vi "Read ballPossession.vi"(8 "error in (no error)":errorcluster, 11 "Events in":refnum<class "Events.lvclass">) -> (0 "error out":errorcluster, 2 "Enum":T1, 3 "Events out":refnum<class "Events.lvclass">)   [LabVIEW 2023, in "Events.lvclass"]
uses:
  Events.lvclass
  Possession.ctl
  Events.lvclass/Events.ctl
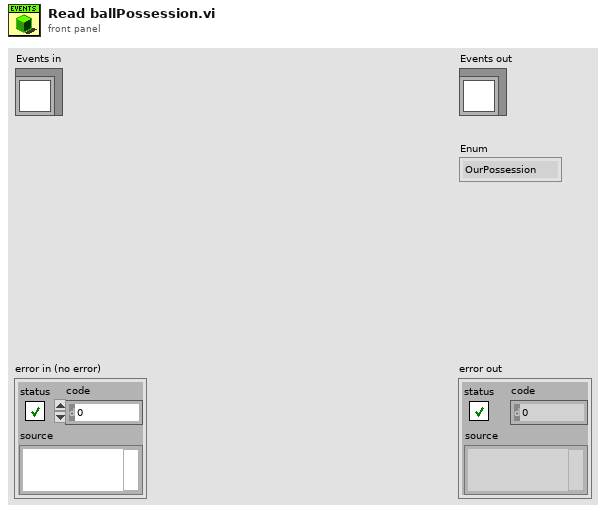
[diagram p1: front panel]
types:
  T1 = typedef "Events.lvclass/Possession.ctl" = enum16{"OurPossession", "TheirPossession", "Contended", "Loose"}
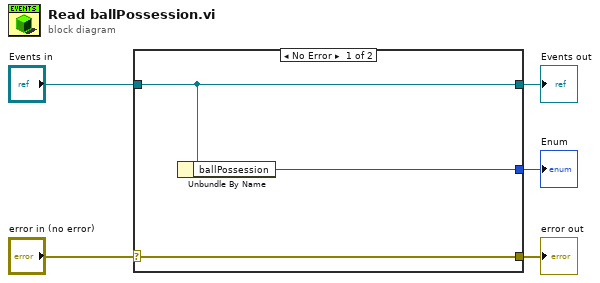
[diagram p0: block diagram]
diagram:
  n1 = case shown="No Error" "error in (no error)" {
    selector: "error in (no error)" -> [w8 w9]
    tunnel: [w8 w9] -> w4
    tunnel: [w7 w10] -> w2
    tunnel: "Events in" -> [w7 w10]
    tunnel: [w6 _] -> w1
    frame No Error {
      n2 = Unbundle By Name(w7) -> ("ballPossession"=w6:T1)
    }
    frame Error {
    }
  }
  "error out" <- w4
  "Events out" <- w2
  "Enum" <- w1
